vi "Main.vi"() -> ()   [LabVIEW 2021]
uses:
  Controls/Pages.ctl
  Controls/ManualTestParameters.ctl
  Controls/AutomaticalTestParameters.ctl
  <vilib>/express/express analysis/Spectral/Block/exnSpectralBlock spectral measurements power poly.vi
  <vilib>/express/express analysis/Spectral/Block/exnSpectralBlock spectral measurements power DDT.vi
  <vilib>/Utility/file.llb/Write Delimited Spreadsheet (string).vi
  <vilib>/express/express analysis/Spectral/XNode/ExpressSpectralMeasurementsBlockNode.xnode
panel:
  in  "Tab Control":T1
  in  "Manual Stop":bool
  in  "Manual Start":bool
  out "REVO. Alternate":dbl
  out "Manual Deflection":dbl
  out "BEND. Moment":dbl
  out "Tachometer":dbl
  in  "Order Open":bool
  in  "Auto Open":bool
  in  "Drive Up":bool
  in  "Drive Down":bool
  in  "Lamp On":bool
  in  "Lamp Off":bool
  out "Power Spectrum":dynamicdata(graph)
  out "Deflection":dbl[](graph)
  in  "Reso Start":bool
  in  "Reso Stop":bool
  out "EstimatedTime_Value":dbl format="%#_3g"
  in  "Auto Stop":bool
  out "Deflection_Value":dbl
  in  "Deflection_Setting":dbl
  out "Cycles_Value":dbl
  in  "Cycles_Setting":dbl
  out "BEND. Moment_Value":dbl
  in  "BEND. Moment_Setting":dbl
  out "Tachometer_Value":dbl
  in  "Tachometer_Setting":dbl
  out "Machine STA.":string
  in  "Auto Start":bool
  in  "Table":string[][](table)
  in  "Save Button":bool
  # "輪圈彎曲力矩耐久測試機"
  # "CORNERING BENDING ENDURANCE TESTER"
  # "金嵩盛機械股份有限公司承製"
  # "King Swen Sheng Machinery Co, Ltd."
  # "FAX: 886-3-4561597"
  # "TEL: 886-3-4384699"
  # "手動測試"
  # "Manual Test"
  # "迴轉轉速/Tachometer:"
  # "RPM"
  # "彎曲力矩/BEND. Moment:"
  # "N．m"
  # "負載偏移量/Deflection:"
  # "mm"
  # "主軸間距/REVO. Alternate:"
  # "M/M"
  # "共振測試"
  # "Resonance Test"
  # "自動測試"
  # "Automatical Test"
  # "機台狀況/Machine STA. :"
  # "設定值/Setting"
  # "實際值/Value"
  # "迴轉轉速/Tachometer:"
  # "RPM"
  # "力矩/BEND. Moment:"
  # "N．m"
  # "圈數/INT. Cycles:"
  # "圈"
  # "偏移量/Deflection:"
  # "mm"
  # "預計完成時間/Estimated Finish Time:"
  # "mins"
  # "報告產生"
  # "Report Generation"
  # "輪圈彎曲力矩耐久測試機"
  # "CORNERING BENDING ENDURANCE TESTER"
  # "金嵩盛機械股份有限公司承製"
  # "King Swen Sheng Machinery Co, Ltd."
  # "FAX: 886-3-4561597"
  # "TEL: 886-3-4384699"
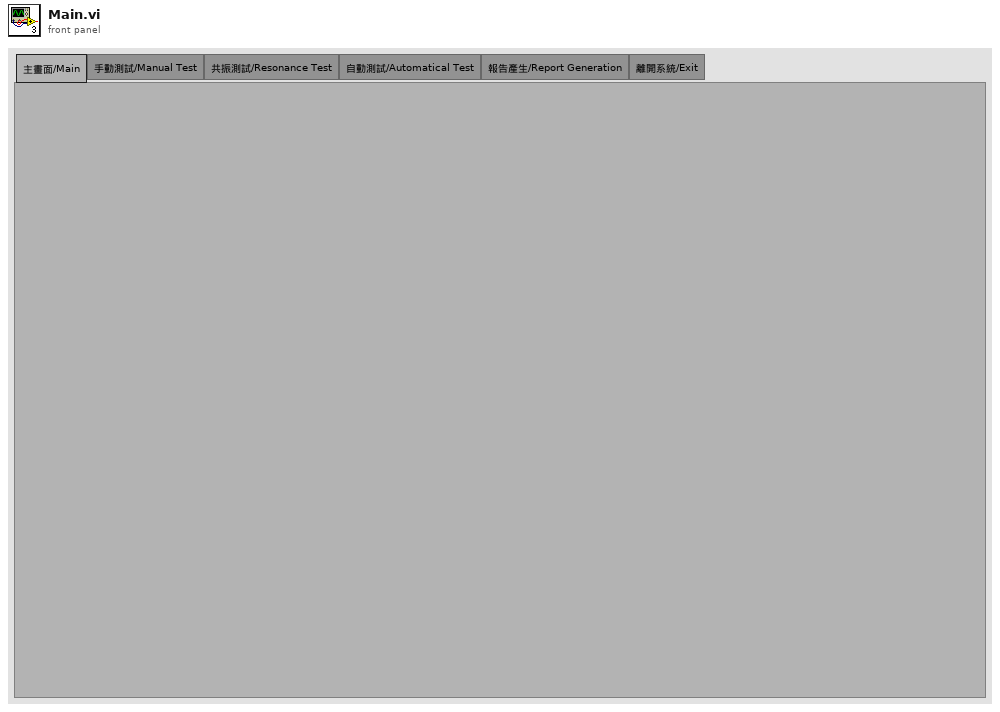
[diagram p1: front panel]
types:
  T1 = typedef "Pages.ctl" = enum32{"主畫面/Main", "手動測試/Manual Test", "共振測試/Resonance Test", "自動測試/Automatical Test", "報告產生/Report Generation", "離開系統/Exit"}
  T2 = typedef "AutomaticalTestParameters.ctl" = cluster{"Machine STA.":string, "Tachometer_Setting":dbl, "BEND. Moment_Setting":dbl, "Cycles_Setting":dbl, "Deflection_Setting":dbl, "Tachometer_Value":dbl, "BEND. Moment_Value":dbl, "Cycles_Value":dbl, "Deflection_Value":dbl, "EstimatedTime_Value":dbl, "Play Button":bool, "Stop Button":bool}
  T3 = typedef "ManualTestParameters.ctl" = cluster{"Order Open":bool, "Auto Open":bool, "Drive Up":bool, "Drive Down":bool, "Lamp On":bool, "Lamp Off":bool, "Tachometer":dbl, "BEND. Moment":dbl, "Deflection":dbl, "REVO. Alternate":dbl, "Drive Up Limit":dbl}
  T4 = cluster{"averaging mode":u16, "weighting mode":u16, "number of averages":u32}
  T5 = cluster{"dB On (F)":bool, "unwrap phase (F)":bool, "convert to degree (F)":bool}
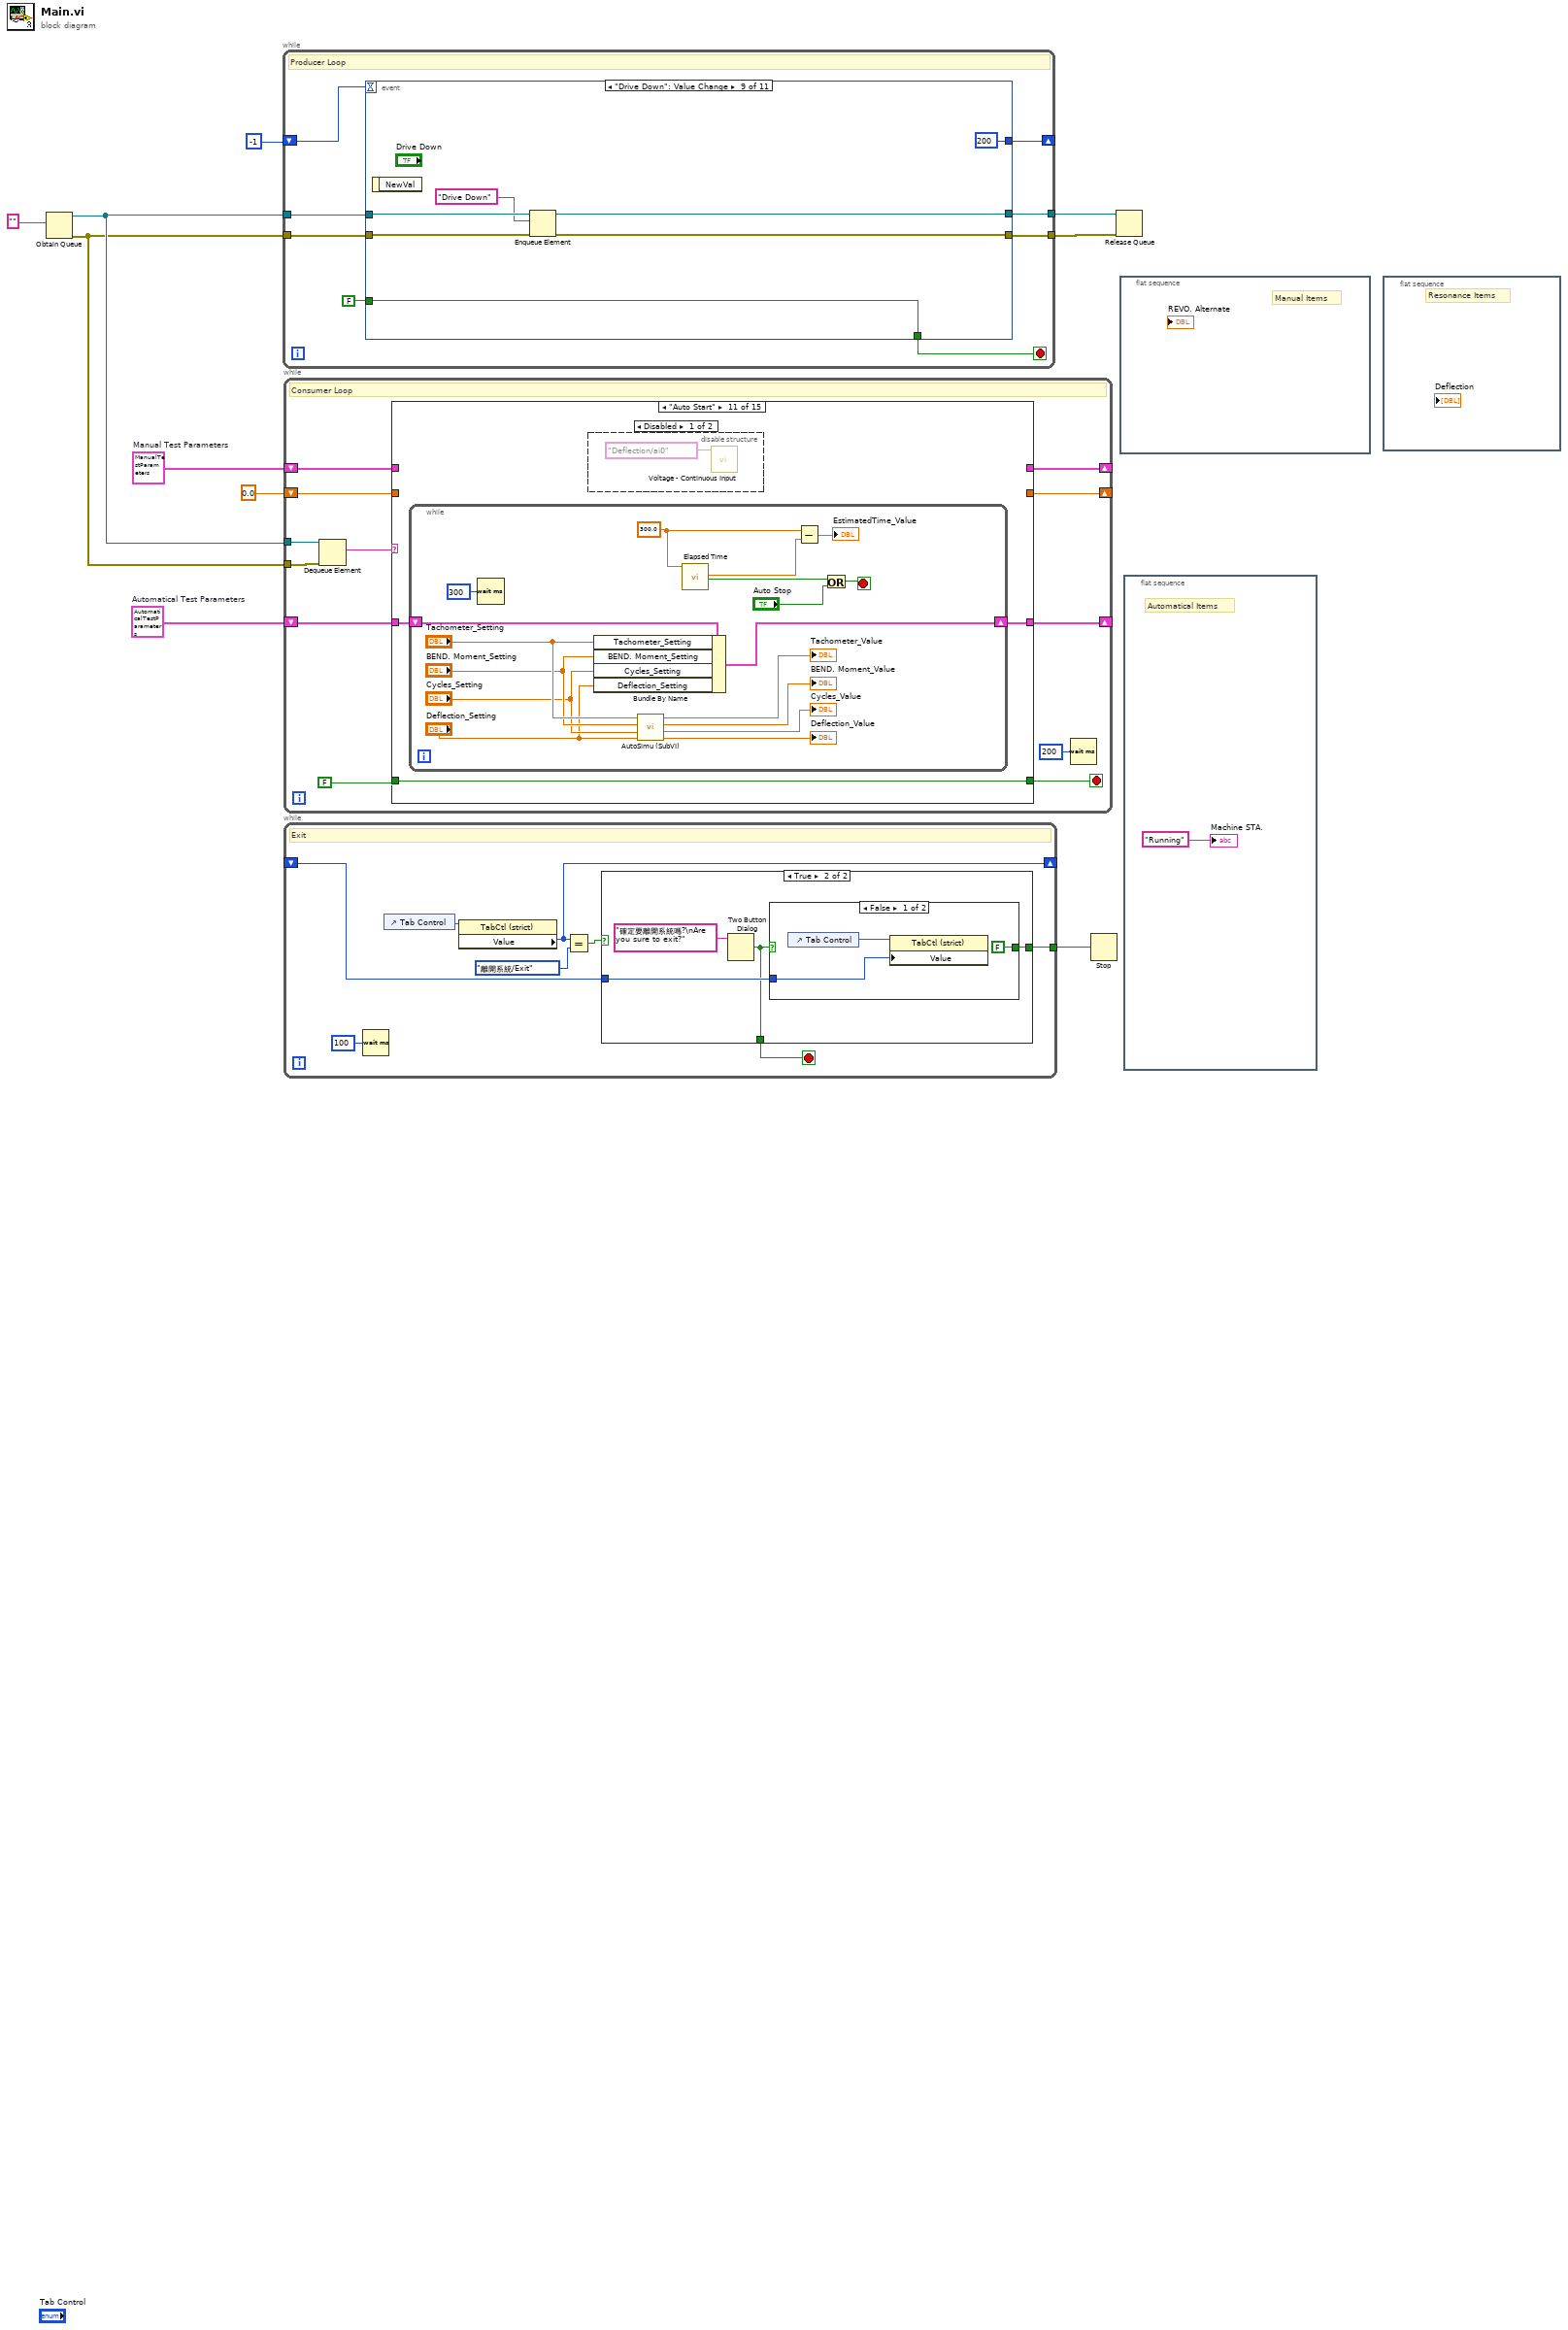
[diagram p0: block diagram]
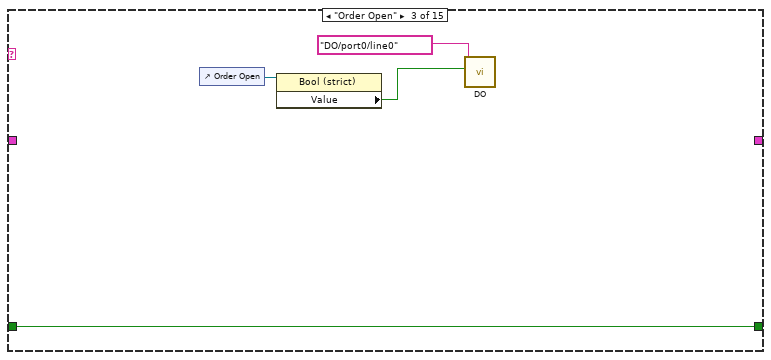
[diagram p4: hidden frame]
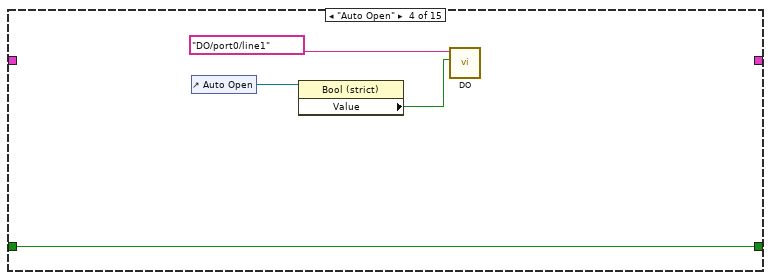
[diagram p5: hidden frame]
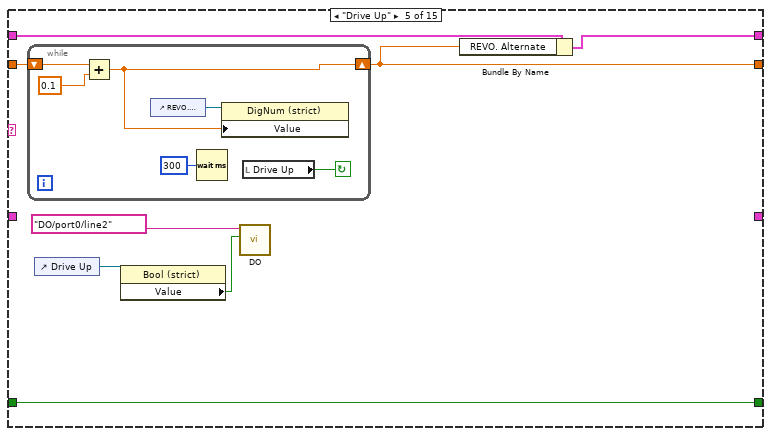
[diagram p6: hidden frame]
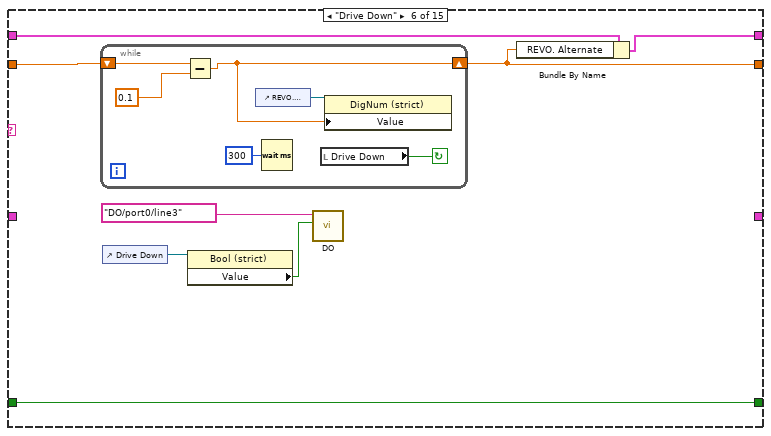
[diagram p7: hidden frame]
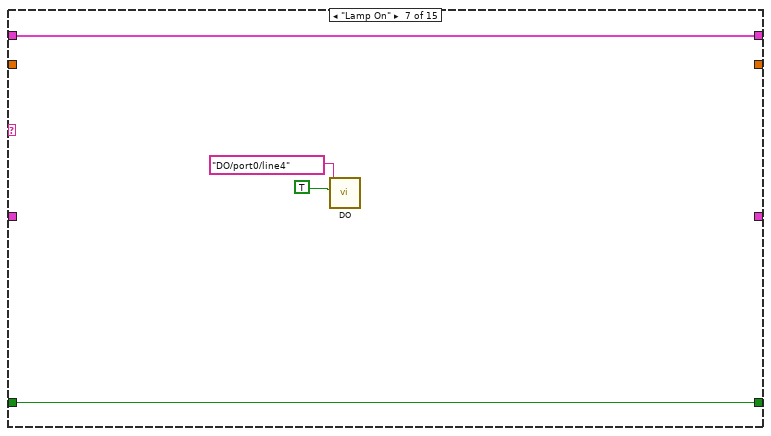
[diagram p8: hidden frame]
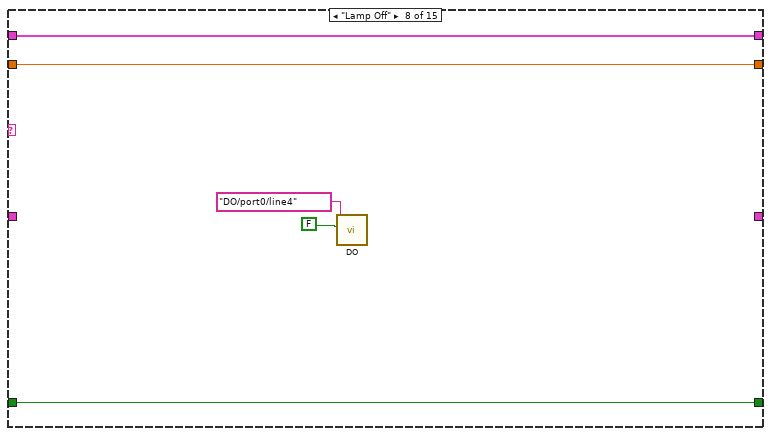
[diagram p9: hidden frame]
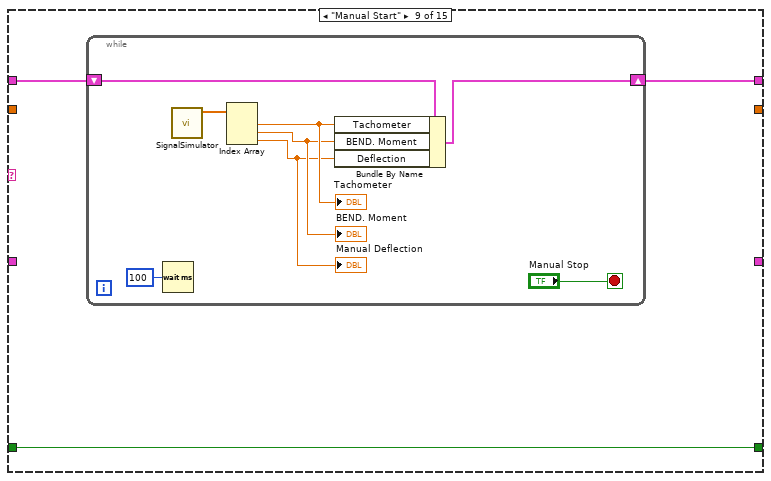
[diagram p10: hidden frame]
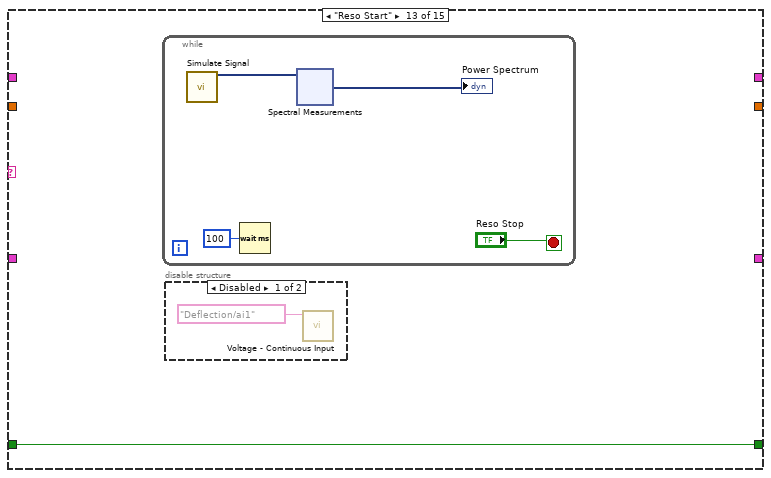
[diagram p14: hidden frame]
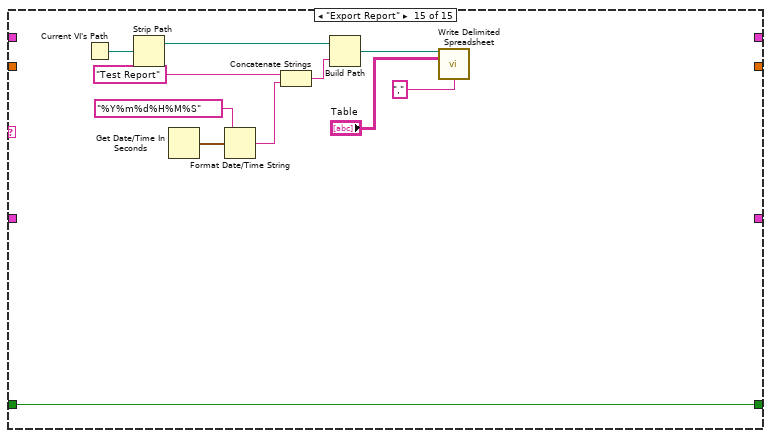
[diagram p17: hidden frame]
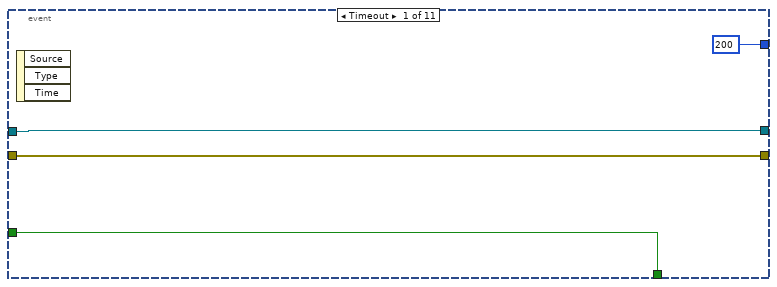
[diagram p18: hidden frame]
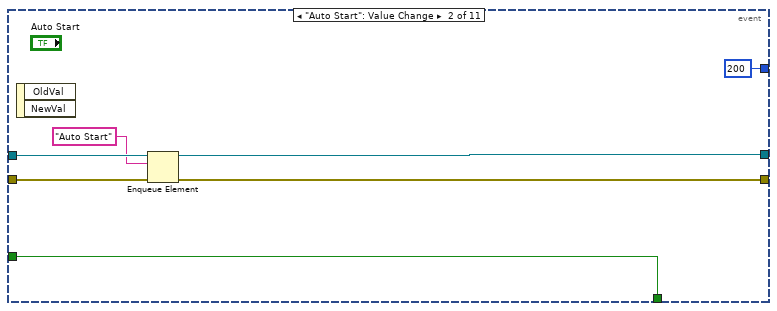
[diagram p19: hidden frame]
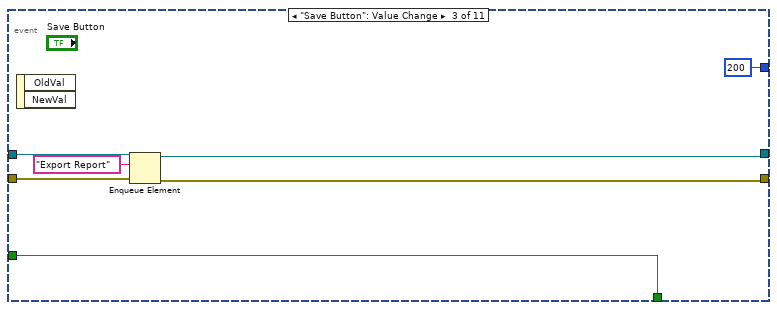
[diagram p20: hidden frame]
diagram:
  w1 = T2 {"Machine STA."="", "Tachometer_Setting"=0.0, "BEND. Moment_Setting"=0.0, "Cycles_Setting"=0.0, "Deflection_Setting"=0.0, "Tachometer_Value"=0.0, "BEND. Moment_Value"=0.0, "Cycles_Value"=0.0, "Deflection_Value"=0.0, "EstimatedTime_Value"=0.0, "Play Button"=FALSE, "Stop Button"=FALSE}  # Automatical Test Parameters
  w3 = T3 {"Order Open"=FALSE, "Auto Open"=FALSE, "Drive Up"=FALSE, "Drive Down"=FALSE, "Lamp On"=FALSE, "Lamp Off"=FALSE, "Tachometer"=0.0, "BEND. Moment"=0.0, "Deflection"=0.0, "REVO. Alternate"=0.0, "Drive Up Limit"=0.0}  # Manual Test Parameters
  n1 = Obtain Queue(element data type="") -> (queue out=w8:refnum<queue>, error out=w7:errorcluster)  [unwired: 4 in, 1 out]
  n2 = while {
    tunnel: w8 -> [w18]
    tunnel: w7 -> [w17]
    tunnel: [w16] -> w6
    tunnel: [w15] -> w5
    shift-right: [w12] -> _
    shift-left: -1 -> [w11]
    stop <- w14 stop-if-true
    # "Producer Loop"
    n3 = event shown="[8] \"Drive Down\": Value Change" {
      selector: _ -> [_ _ _ _ _ _ _ _ _ _ _]
      dyn-events: _ -> [_ _ _ _ _ _ _ _ _ _ _]
      timeout: w11 -> [_ _ _ _ _ _ _ _ _ _ _]
      tunnel: w18 -> [w22 w29 w36 w43 w50 w57 w64 w71 w78 w85 w92]
      tunnel: w17 -> [w21 w28 w35 w42 w49 w56 w63 w70 w77 w84 w91]
      tunnel: [w22 w27 w34 w41 w47 w53 w61 w69 w75 w82 w89] -> w16
      tunnel: [w21 w26 w33 w40 w46 w52 w60 w68 w74 w81 w88] -> w15
      tunnel: [w20 w23 w30 w37 w45 w55 w59 w66 w73 w80 w87] -> w14
      tunnel: FALSE -> [w20 w23 w30 w37 w45 w55 w59 w66 w73 w80 w87]
      tunnel: [200 200 200 200 200 200 200 200 200 200 200] -> w12
      event Timeout {
        n4 = event-data() -> ()  [unwired: 1 in, 3 out]
      }
      event "Auto Start": Value Change {
        n5 = event-data() -> ()  [unwired: 1 in, 2 out]
        n6 = Enqueue Element(queue=w29, element="Auto Start", error in (no error)=w28) -> (queue out=w27:refnum<queue>, error out=w26:errorcluster)  [unwired: 1 in, 1 out]
      }
      event "Save Button": Value Change {
        n7 = event-data() -> ()  [unwired: 1 in, 2 out]
        n8 = Enqueue Element(queue=w36, element="Export Report", error in (no error)=w35) -> (queue out=w34:refnum<queue>, error out=w33:errorcluster)  [unwired: 1 in, 1 out]
      }
      event "Reso Start": Value Change {
        n9 = event-data() -> ()  [unwired: 1 in, 2 out]
        n10 = Enqueue Element(queue=w43, element="Reso Start", error in (no error)=w42) -> (queue out=w41:refnum<queue>, error out=w40:errorcluster)  [unwired: 1 in, 1 out]
      }
      event "Order Open": Value Change {
        n11 = event-data() -> ()  [unwired: 1 in, 1 out]
        n12 = Enqueue Element(queue=w50, element="Order Open", error in (no error)=w49) -> (queue out=w47:refnum<queue>, error out=w46:errorcluster)  [unwired: 1 in, 1 out]
      }
      event "Manual Start": Value Change {
        n13 = event-data() -> ()  [unwired: 1 in, 1 out]
        n14 = Enqueue Element(queue=w57, element="Manual Start", error in (no error)=w56) -> (queue out=w53:refnum<queue>, error out=w52:errorcluster)  [unwired: 1 in, 1 out]
      }
      event "Auto Open": Value Change {
        n15 = event-data() -> ()  [unwired: 1 in, 1 out]
        n16 = Enqueue Element(queue=w64, element="Auto Open", error in (no error)=w63) -> (queue out=w61:refnum<queue>, error out=w60:errorcluster)  [unwired: 1 in, 1 out]
      }
      event "Drive Up": Value Change {
        n17 = event-data() -> ()  [unwired: 1 in, 1 out]
        n18 = Enqueue Element(queue=w71, element="Drive Up", error in (no error)=w70) -> (queue out=w69:refnum<queue>, error out=w68:errorcluster)  [unwired: 1 in, 1 out]
      }
      event "Drive Down": Value Change {
        n19 = event-data() -> ()  [unwired: 1 in, 1 out]
        n20 = Enqueue Element(queue=w78, element="Drive Down", error in (no error)=w77) -> (queue out=w75:refnum<queue>, error out=w74:errorcluster)  [unwired: 1 in, 1 out]
      }
      event "Lamp On": Value Change {
        n21 = event-data() -> ()  [unwired: 1 in, 1 out]
        n22 = Enqueue Element(queue=w85, element="Lamp On", error in (no error)=w84) -> (queue out=w82:refnum<queue>, error out=w81:errorcluster)  [unwired: 1 in, 1 out]
      }
      event "Lamp Off": Value Change {
        n23 = event-data() -> ()  [unwired: 1 in, 1 out]
        n24 = Enqueue Element(queue=w92, element="Lamp Off", error in (no error)=w91) -> (queue out=w89:refnum<queue>, error out=w88:errorcluster)  [unwired: 1 in, 1 out]
      }
    }
  }
  n25 = while {
    tunnel: w8 -> [w104]
    tunnel: w7 -> [w103]
    shift-right: [w98] -> _
    shift-left: w3 -> [w99]
    shift-right: [w96] -> _
    shift-left: 0.0 -> [w97]
    shift-right: [w93] -> _
    shift-left: w1 -> [w94]
    stop <- w101 stop-if-true
    # "Consumer Loop"
    n26 = Dequeue Element(queue=w104, error in (no error)=w103) -> (element=w102:string)  [unwired: 1 in, 3 out]
    n27 = case shown="\"Auto Start\"" w102 {
      tunnel: [w105 w106 w110 w114 w122 w136 w146 w151 w154 w165 w168 w187 w188 w203 w214] -> w101
      tunnel: FALSE -> [w105 w106 w110 w114 w122 w136 w146 w151 w154 w165 w168 w187 w188 w203 w214]
      tunnel: w99 -> [_ _ _ _ w118 w132 w143 w148 w153 w164 _ _ _ _ _]
      tunnel: [_ _ _ _ w116 w131 w143 w148 w152 w164 _ _ _ _ _] -> w98
      tunnel: w97 -> [_ _ _ _ w117 w130 _ w147 _ w163 _ _ _ _ _]
      tunnel: [_ _ _ _ w115 w129 _ w147 _ w163 _ _ _ _ _] -> w96
      tunnel: w94 -> [_ _ _ _ _ _ _ _ _ _ w167 _ _ _ _]
      tunnel: [_ _ _ _ _ _ _ _ _ _ w166 _ _ _ _] -> w93
      frame "False", Default {
      }
      frame "-----Manual Test-----" {
      }
      frame "Order Open" {
        n28 = control-ref of="Order Open"() -> (w108:refnum<vi>)
        n29 = property class="Bool (strict)"(reference=w108) -> ("Value"=w107:bool)  [unwired: 1 in, 2 out]
        n30 = call "DO.vi"("data"=w107, "Line(s)"=tag "DO/port0/line0") -> ()  [unwired: 9 in, 1 out]
      }
      frame "Auto Open" {
        n31 = control-ref of="Auto Open"() -> (w112:refnum<vi>)
        n32 = property class="Bool (strict)"(reference=w112) -> ("Value"=w111:bool)  [unwired: 1 in, 2 out]
        n33 = call "DO.vi"("data"=w111, "Line(s)"=tag "DO/port0/line1") -> ()  [unwired: 9 in, 1 out]
      }
      frame "Drive Up" {
        n34 = while {
          shift-right: [w123] -> w115
          shift-left: w117 -> [w128]
          stop <- w126 continue-if-true
          n35 = Add(x=w128, y=0.1) -> (x+y=w123:dbl)
          n36 = control-ref of="REVO. Alternate"() -> (w124:refnum<vi>)
          n37 = Wait (ms)(milliseconds to wait=u32 300) -> ()  [unwired: 1 out]
          n38 = property class="DigNum (strict)"(reference=w124, "Value"=w123) -> ()  [unwired: 1 in, 2 out]
          n39 = local read "Drive Up"() -> (w126:bool)
        }
        n40 = control-ref of="Drive Up"() -> (w120:refnum<vi>)
        n41 = property class="Bool (strict)"(reference=w120) -> ("Value"=w119:bool)  [unwired: 1 in, 2 out]
        n42 = call "DO.vi"("data"=w119, "Line(s)"=tag "DO/port0/line2") -> ()  [unwired: 9 in, 1 out]
        n43 = Bundle By Name(cluster=w118, "REVO. Alternate"=w115) -> (w116:T3)
      }
      frame "Drive Down" {
        n44 = while {
          shift-right: [w139] -> w129
          shift-left: w130 -> [w141]
          stop <- w138 continue-if-true
          n45 = Subtract(x=w141, y=0.1) -> (x-y=w139:dbl)
          n46 = control-ref of="REVO. Alternate"() -> (w140:refnum<vi>)
          n47 = Wait (ms)(milliseconds to wait=u32 300) -> ()  [unwired: 1 out]
          n48 = local read "Drive Down"() -> (w138:bool)
          n49 = property class="DigNum (strict)"(reference=w140, "Value"=w139) -> ()  [unwired: 1 in, 2 out]
        }
        n50 = control-ref of="Drive Down"() -> (w134:refnum<vi>)
        n51 = property class="Bool (strict)"(reference=w134) -> ("Value"=w133:bool)  [unwired: 1 in, 2 out]
        n52 = call "DO.vi"("data"=w133, "Line(s)"=tag "DO/port0/line3") -> ()  [unwired: 9 in, 1 out]
        n53 = Bundle By Name(cluster=w132, "REVO. Alternate"=w129) -> (w131:T3)
      }
      frame "Lamp On" {
        n54 = call "DO.vi"("data"=TRUE, "Line(s)"=tag "DO/port0/line4") -> ()  [unwired: 9 in, 1 out]
      }
      frame "Lamp Off" {
        n55 = call "DO.vi"("data"=FALSE, "Line(s)"=tag "DO/port0/line4") -> ()  [unwired: 9 in, 1 out]
      }
      frame "Manual Start" {
        n56 = while {
          shift-right: [w158] -> w152
          shift-left: w153 -> [w160]
          stop <- "Manual Stop" stop-if-true
          n57 = Wait (ms)(milliseconds to wait=u32 100) -> ()  [unwired: 1 out]
          n58 = call "SignalSimulator.vi"() -> ("Array"=w162:dbl[])  [unwired: 11 in]
          n59 = Index Array(array=w162) -> (element #1=w157:dbl, element #2=w156:dbl, element #3=w155:dbl)  [unwired: 3 in]
          "Tachometer" <- w157
          "BEND. Moment" <- w156
          "Manual Deflection" <- w155
          n60 = Bundle By Name(cluster=w160, "Tachometer"=w157, "BEND. Moment"=w156, "Deflection"=w155) -> (w158:T3)
        }
      }
      frame "-----Automatical Test-----" {
      }
      frame "Auto Start" {
        n61 = while {
          shift-right: [w185] -> w166
          shift-left: w167 -> [w186]
          stop <- w175 stop-if-true
          w174 = 300.0 ("Time Target (s)")
          n62 = Wait (ms)(milliseconds to wait=u32 300) -> ()  [unwired: 1 out]
          n63 = Bundle By Name(cluster=w186, "Tachometer_Setting"="Tachometer_Setting", "BEND. Moment_Setting"="BEND. Moment_Setting", "Cycles_Setting"="Cycles_Setting", "Deflection_Setting"="Deflection_Setting") -> (w185:T2)
          n64 = call "AutoSimu (SubVI).vi"("Deflection_Setting 5"="Deflection_Setting", "Cycles_Setting"="Cycles_Setting", "BEND. Moment_Setting"="BEND. Moment_Setting", "Tachometer_Setting"="Tachometer_Setting") -> ("Deflection_Setting"=→"Deflection_Value":dbl, "Deflection_Setting 2"=→"Cycles_Value":dbl, "Deflection_Setting 3"=→"BEND. Moment_Value":dbl, "Deflection_Setting 4"=→"Tachometer_Value":dbl)  [unwired: 4 in]
          n65 = call "Elapsed Time"("Time Target (s)"=w174) -> ("Elapsed Time (s)"=w173:dbl, "Time has Elapsed"=w177:bool)  [unwired: 11 in, 6 out]
          n66 = Subtract(x=w174, y=w173) -> (x-y=→"EstimatedTime_Value":dbl)
          n67 = Or(x=w177, y="Auto Stop") -> (x .or. y?=w175:bool)
        }
        n68 = disable-structure shown="Disabled" {
          frame Disabled {
            n69 = call "Voltage - Continuous Input.vi"("Physical Channel"=tag "Deflection/ai0") -> ()  [unwired: 9 in, 2 out]
          }
          frame Enabled {
          }
        }
      }
      frame "-----Resonance Test-----" {
      }
      frame "Reso Start" {
        n70 = while {
          stop <- "Reso Stop" stop-if-true
          n71 = call "Simulate Signal"() -> ("Sine"=w190:dynamicdata)  [unwired: 14 in, 1 out]
          n72 = Wait (ms)(milliseconds to wait=u32 100) -> ()  [unwired: 1 out]
          n73 = xnode "Spectral Measurements"("Signals"=w190) -> ("Power Spectrum"=→"Power Spectrum":dynamicdata)  [unwired: 1 in, 1 out]
        }
        n74 = disable-structure shown="Disabled" {
          frame Disabled {
            n75 = call "Voltage - Continuous Input.vi"("Physical Channel"=tag "Deflection/ai1") -> ()  [unwired: 9 in, 2 out]
          }
          frame Enabled {
          }
        }
      }
      frame "-----Report Generation-----" {
      }
      frame "Export Report" {
        n76 = Current VI's Path() -> (path=w212:path)
        n77 = Strip Path(path=w212) -> (stripped path=w210:path)  [unwired: 1 out]
        n78 = Get Date/Time In Seconds() -> (seconds since 1Jan1904=w209:timestamp)
        n79 = Format Date/Time String(time format string (%c)="%Y%m%d%H%M%S", seconds (now)=w209) -> (date/time string=w205:string)  [unwired: 1 in]
        n80 = Concatenate Strings("Test Report" ("string"), w205) -> (w207:string)
        n81 = Build Path(base path=w210, name or relative path=w207) -> (appended path=w211:path)
        n82 = call-poly <vilib>:"Write Delimited Spreadsheet.vi"("file path (dialog if empty)"=w211, "2D data"="Table", "delimiter (\\t)"="," ("delimiter (\\t)")) -> ()  [unwired: 11 in, 2 out]
      }
    }
    n83 = Wait (ms)(milliseconds to wait=u32 200) -> ()  [unwired: 1 out]
  }
  n84 = while {
    tunnel: [w219] -> w10
    shift-right: [w218] -> _
    shift-left: _ -> [w217]
    stop <- w216 stop-if-true
    # "Exit"
    n85 = Wait (ms)(milliseconds to wait=u32 100) -> ()  [unwired: 1 out]
    n86 = control-ref of="Tab Control"() -> (w222:refnum<vi>)
    n87 = property class="TabCtl (strict)"(reference=w222) -> ("Value"=w218:T1)  [unwired: 1 in, 2 out]
    n88 = Equal?(x=w218, y=Pages."離開系統/Exit") -> (x = y?=w220:bool)
    n89 = case shown="True" w220 {
      tunnel: [FALSE w227] -> w219
      tunnel: w217 -> [_ w226]
      tunnel: [FALSE ("T button?") w225] -> w216
      frame False {
      }
      frame True {
        n90 = Two Button Dialog(message="確定要離開系統嗎?\nAre you sure to exit?") -> (T button?=w225:bool)  [unwired: 2 in]
        n91 = case shown="False" w225 {
          selector: w225 -> [_ w232]
          tunnel: [FALSE w232] -> w227
          tunnel: w226 -> [w229 _]
          frame False {
            n92 = control-ref of="Tab Control"() -> (w231:refnum<vi>)
            n93 = property class="TabCtl (strict)"(reference=w231, "Value"=w229) -> ()  [unwired: 1 in, 2 out]
          }
          frame True {
          }
        }
      }
    }
  }
  n94 = Stop(stop? (T)=w10) -> ()
  n95 = Release Queue(queue=w6, error in (no error)=w5) -> ()  [unwired: 1 in, 3 out]
  n96 = flat-sequence {
    frame #0 {
      # "Manual Items"
    }
  }
  n97 = flat-sequence {
    frame #0 {
      # "Automatical Items"
      "Machine STA." <- "Running" ("Machine STA.")
    }
  }
  n98 = flat-sequence {
    frame #0 {
      # "Resonance Items"
    }
  }
